vi "Wait.Gui.UpdateProgBar.vi"(8 "error in (no error)":errorcluster, 9 "ProgBar (0)":i32, 10 "status (\"\")":string) -> (0 "error out":errorcluster)   [LabVIEW 2016]
uses:
  Wait.Gui.Action.ctl
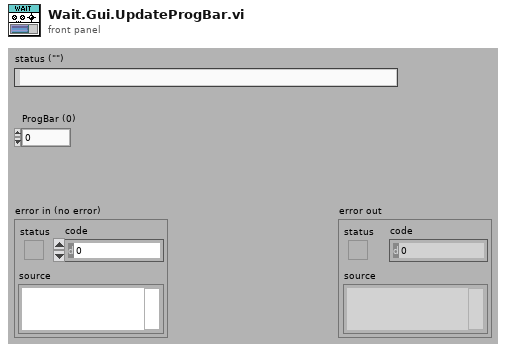
[diagram p1: front panel]
types:
  T1 = typedef "Wait.Gui.Action.ctl" = enum32{"idle", "constructor", "destructor", "--- WaitGui ---", "open FP", "close FP", "update msg", "update progbar"}
  T2 = cluster{"status (\"\")":string, "ProgBar (0)":i32}
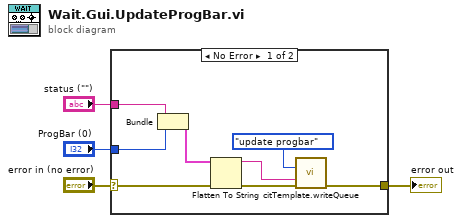
[diagram p0: block diagram]
diagram:
  n1 = case shown="No Error" "error in (no error)" {
    selector: "error in (no error)" -> [w8 w13]
    tunnel: [w12 w13] -> w4
    tunnel: "ProgBar (0)" -> [w6 _]
    tunnel: "status (\"\")" -> [w7 _]
    frame No Error {
      n2 = Bundle("status (\"\")"=w7, "ProgBar (0)"=w6) -> (w5:T2)  [unwired: 1 in]
      n3 = Flatten To String(anything=w5, error in (no error)=w8) -> (data string=w10:string, error out=w9:errorcluster)  [unwired: 2 in, 1 out]
      n4 = call "citTemplate.writeQueue.vi"("event in (if not connected:all statemachine with data event)"=Wait.Gui.Action."update progbar" ("Action"), "data in"=w10, "error in (no error)"=w9) -> ("error out"=w12:errorcluster)  [unwired: 12 in]
    }
    frame Error {
    }
  }
  "error out" <- w4
